vi "Add Round Key2.vi"(7 "Nb":i32=4, 8 "error in":errorcluster, 9 "rnd (0)":i32, 10 "State.In":u16[][](array[numeric]), 11 "ExpandedKey(w)":u32[][](array[numeric])) -> (0 "error out":errorcluster, 2 "State.Out":u16[][](array[numeric]))   [LabVIEW 2016, in "数据传输系统-06.lvlib"]
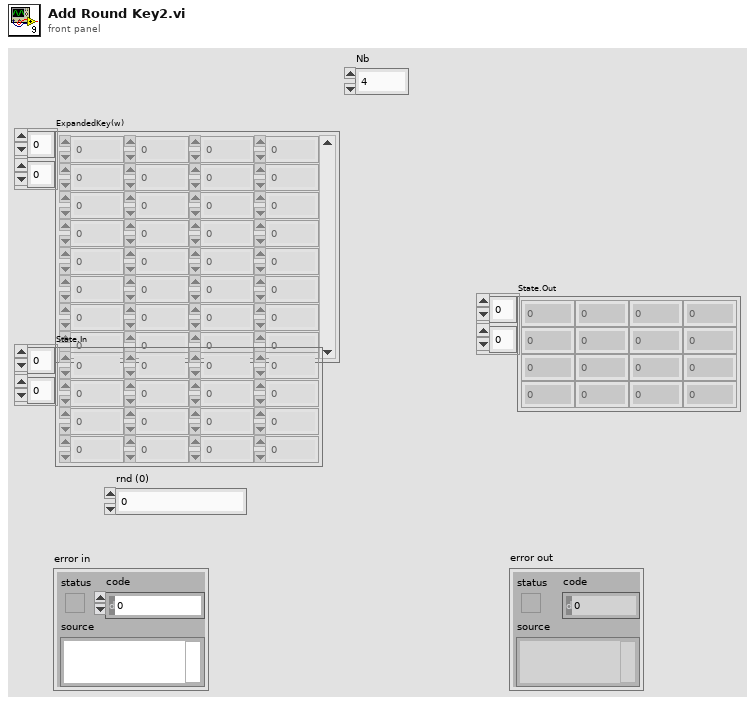
[diagram p1: front panel]
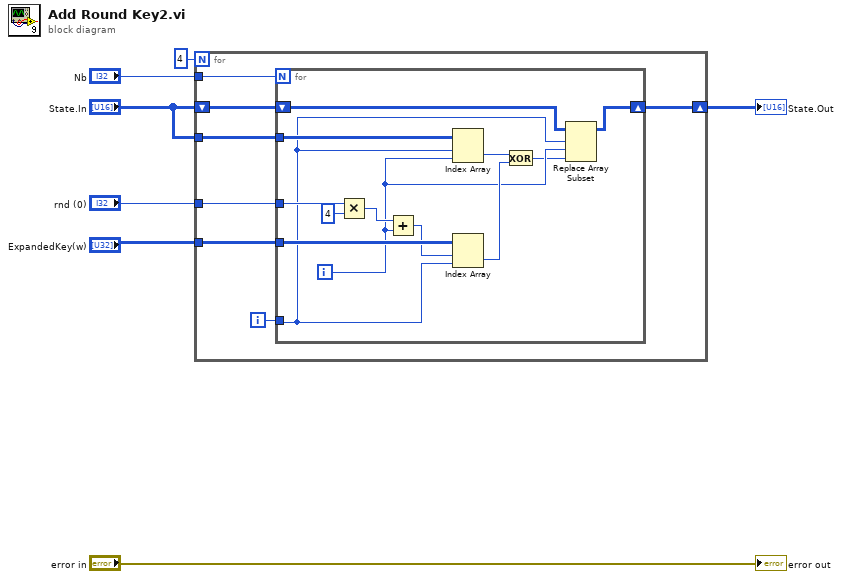
[diagram p0: block diagram]
diagram:
  n1 = for {
    N: 4 -> [_]
    tunnel: "State.In" -> [w13]
    tunnel: "ExpandedKey(w)" -> [w12]
    tunnel: "Nb" -> [w11]
    tunnel: "rnd (0)" -> [w10]
    shift-right: [w8] -> w2
    shift-left: "State.In" -> [w9]
    i -> [w14]
    n2 = for {
      N: w11 -> [_]
      tunnel: w14 -> [w19]
      tunnel: w13 -> [w22]
      tunnel: w12 -> [w27]
      tunnel: w10 -> [w26]
      shift-right: [w15] -> w8
      shift-left: w9 -> [w16]
      i -> [w18]
      n3 = Multiply(x=w26, y=4) -> (x*y=w24:i32)
      n4 = Add(x=w24, y=w18) -> (x+y=w23:i32)
      n5 = Index Array(array=w22, index (row)=w19, index (col)=w18) -> (element=w21:u16)
      n6 = Index Array(array=w27, index (row)=w23, index (col)=w19) -> (element=w20:u32)
      n7 = Exclusive Or(1:w20, 2:w21) -> (0:w17:u32)
      n8 = Replace Array Subset(array=w16, new element=w17, index (row)=w19, index (col)=w18) -> (w15:u16[][])
    }
  }
  "State.Out" <- w2
  "error out" <- "error in"
